vi "set_clock.vi"(8 "error in (no error)":errorcluster, 10 "clock":refnum<class "GenericClock.lvclass">, 11 "Stimulator090724Scaffold in":refnum<class "Stimulator090724Scaffold.lvclass">) -> (0 "error out":errorcluster, 3 "Stimulator090724Scaffold out":refnum<class "Stimulator090724Scaffold.lvclass">)   [LabVIEW 2010]
uses:
  Stimulator090724Scaffold.lvclass
  Clock/GenericClock/GenericClock/GenericClock.lvclass
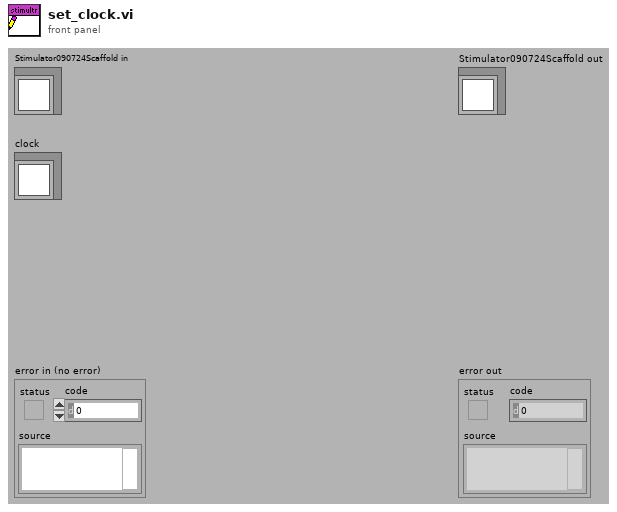
[diagram p1: front panel]
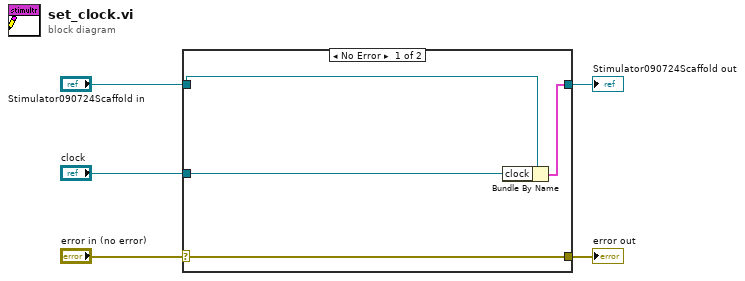
[diagram p0: block diagram]
diagram:
  n1 = case shown="No Error" "error in (no error)" {
    selector: "error in (no error)" -> [w9 w10]
    tunnel: [w9 w10] -> w4
    tunnel: [w7 w11] -> w2
    tunnel: "Stimulator090724Scaffold in" -> [w8 w11]
    tunnel: "clock" -> [w6 _]
    frame No Error {
      n2 = Bundle By Name(cluster=w8, "clock"=w6) -> (w7:cluster{})
    }
    frame Error {
    }
  }
  "error out" <- w4
  "Stimulator090724Scaffold out" <- w2
